vi "Read Arduino Resource.vi"(11 "DAQ in":refnum<class "DAQ.lvclass">) -> (2 "Arduino Resource":T1={"VISA resource"="", "Board Type"=enum."Uno", "Connection Type"=enum."USB / Serial", "Bytes Per Packet (15)"=15}, 3 "DAQ out":refnum<class "DAQ.lvclass">)   [LabVIEW 2011, in "DAQ.lvclass"]
uses:
  DAQ.lvclass
  <vilib>/LabVIEW Interface for Arduino/Type Defs/Arduino Resource.ctl
  <vilib>/LabVIEW Interface for Arduino/Type Defs/Board Type.ctl
  DAQ.lvclass/DAQ.ctl
  <vilib>/LabVIEW Interface for Arduino/LabVIEW Interface for Arduino.lvlib
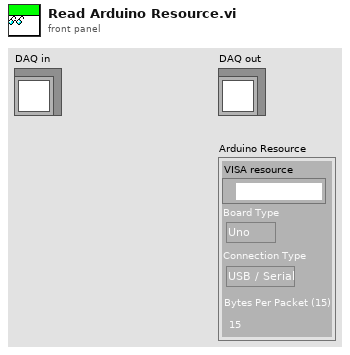
[diagram p1: front panel]
types:
  T1 = typedef "LabVIEW Interface for Arduino.lvlib/Arduino Resource.ctl" = cluster{"VISA resource":refnum<visa-resource-name>, "Board Type":T2, "Connection Type":enum8{"USB / Serial"}, "Bytes Per Packet (15)":u8}
  T2 = typedef "LabVIEW Interface for Arduino.lvlib/Board Type.ctl" = enum16{"Uno", "Dimuelanove w/Atmega 328", "Mega 2560"}
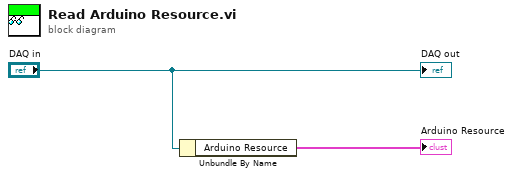
[diagram p0: block diagram]
diagram:
  n1 = Unbundle By Name("DAQ in") -> ("Arduino Resource"=→"Arduino Resource":T1)
  "DAQ out" <- "DAQ in"
